vi "StripComments.vi"(11 "String":string) -> (1 "Keep line":bool, 3 "trimmed string":string)   [LabVIEW 2016]
uses:
  <vilib>/Utility/error.llb/whitespace.ctl
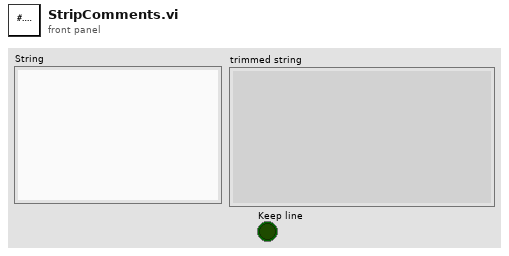
[diagram p1: front panel]
types:
  T1 = typedef "whitespace.ctl" = u16
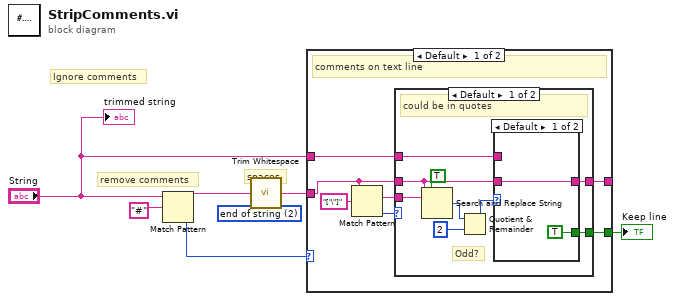
[diagram p0: block diagram]
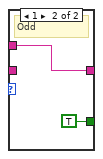
[diagram p2: hidden frame]
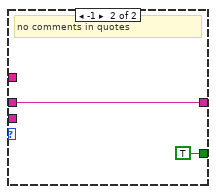
[diagram p3: hidden frame]
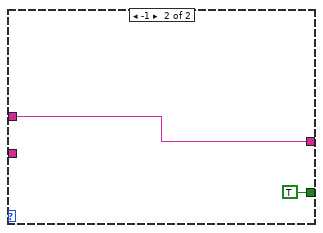
[diagram p4: hidden frame]
diagram:
  w7 = T1 2 items=["both", "start of string", "end of string"] ("location (both)")
  # "Ignore comments"
  # "spaces"
  # "remove comments"
  n1 = Match Pattern(string="String", regular expression="#") -> (before substring=w6:string, offset past match=w3:i32)  [unwired: 1 in, 2 out]
  n2 = call <vilib>:"Trim Whitespace.vi"("string"=w6, "location (both)"=w7) -> ("trimmed string"=w2:string)
  n3 = case shown="Default" w3 {
    tunnel: [w12 w30] -> _
    tunnel: "String" -> [w10 w30]
    tunnel: [w9 TRUE] -> w4
    tunnel: w2 -> [w8 _]
    frame Default {
      # "comments on text line"
      n4 = Match Pattern(string=w8, regular expression="['\"]") -> (match substring=w11:string, offset past match=w13:i32)  [unwired: 1 in, 2 out]
      n5 = case shown="Default" w13 {
        tunnel: [w18 w29] -> w12
        tunnel: w8 -> [w16 w29]
        tunnel: w11 -> [w23 _]
        tunnel: w10 -> [w17 _]
        tunnel: [w15 TRUE] -> w9
        frame Default {
          # "Odd?"
          # "could be in quotes"
          n6 = Search and Replace String(replace all?=TRUE ("replace all? (F)"), input string=w16, search string=w23) -> (number of replacements=w21:i32)  [unwired: 5 in, 3 out]
          n7 = Quotient & Remainder(x=w21, y=2) -> (x-y*floor(x/y)=w19:i32)  [unwired: 1 out]
          n8 = case shown="Default" w19 {
            tunnel: [w25 w27] -> w18
            tunnel: w17 -> [_ w27]
            tunnel: w16 -> [w25 _]
            tunnel: [TRUE TRUE] -> w15
            frame Default {
            }
            frame 1 {
              # "Odd"
            }
          }
        }
        frame -1 {
          # "no comments in quotes"
        }
      }
    }
    frame -1 {
    }
  }
  "Keep line" <- w4
  "trimmed string" <- "String"
